vi "PWM Wing Duty Cycle Calculation.vi"(9 "End Angle Duty Cycle":fxp<+,8,0>, 10 "Start Angle Duty Cycle":fxp<+,8,0>, 11 "Sector":u8) -> (3 "Duty Cycle Out":fxp<+,8,0>)   [LabVIEW 2013]
uses:
  <vilib>/rvi/Analysis/common/FxpNativeNode/niFpgaFxpNative.xnode
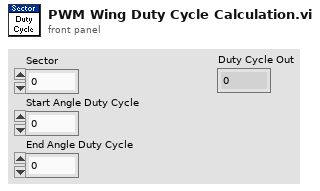
[diagram p1: front panel]
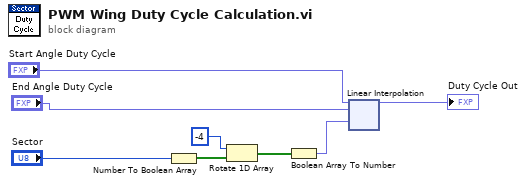
[diagram p0: block diagram]
diagram:
  n1 = Number To Boolean Array(number="Sector") -> (Boolean array=w4:bool[])
  n2 = Rotate 1D Array(1:w4, 2:-4 ("n")) -> (0:w3:bool[])
  n3 = Boolean Array To Number(Boolean array=w3) -> (number=w2:fxp<+,8,0>)
  n4 = xnode ("Linear Interpolation")("y0"="Start Angle Duty Cycle", "y1"="End Angle Duty Cycle", "x"=w2) -> ("y"=→"Duty Cycle Out":fxp<+/-,9,1>)
